vi "joystick_get_pressed.vi"(0 "JoystickDevRef 2":T2, 1 "Scaler":i8=127) -> (2 "JoystickDevRef":T2, 3 "Axes":T1, 4 "Buttons":T4, 5 "Buttons Pressed?":bool[](array[boolean]))   [LabVIEW 2013]
uses:
  <vilib>/Rock Robotics/WPI/Joystick/WPI_JoystickDevRef.ctl
  <vilib>/Rock Robotics/WPI/Joystick/WPI_JoystickDeviceEnum.ctl
  <vilib>/Rock Robotics/WPI/Joystick/WPI_JoystickButtonState.ctl
  <vilib>/Rock Robotics/WPI/Joystick/WPI_JoystickCacheOp.ctl
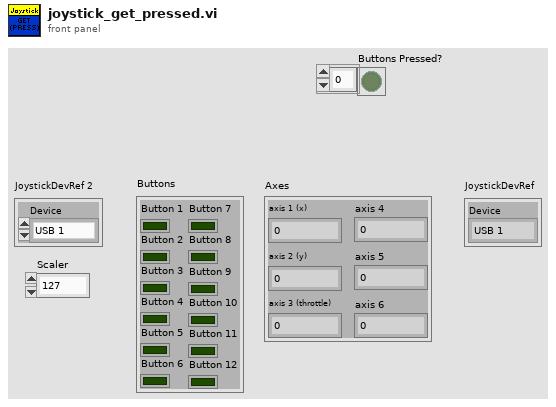
[diagram p1: front panel]
types:
  T1 = cluster{"axis 1 (x)":dbl, "axis 2 (y)":dbl, "axis 3 (throttle)":dbl, "axis 4":dbl, "axis 5":dbl, "axis 6":dbl}
  T2 = typedef "WPI_JoystickDevRef.ctl" = cluster{"Device":T3}
  T3 = typedef "WPI_JoystickDeviceEnum.ctl" = enum16{"USB 1", "USB 2", "USB 3", "USB 4", "Kinect 1", "Kinect 2"}
  T4 = typedef "WPI_JoystickButtonState.ctl" = cluster{"Button 1":bool, "Button 2":bool, "Button 3":bool, "Button 4":bool, "Button 5":bool, "Button 6":bool, "Button 7":bool, "Button 8":bool, "Button 9":bool, "Button 10":bool, "Button 11":bool, "Button 12":bool}
  T5 = cluster{"axis 1 (x)":dbl, "axis 2 (y)":dbl, "axis 3 (z)":dbl, "axis 4 (twist)":dbl, "axis 5 (throttle)":dbl, "axis 6 (num)":dbl}
  T6 = typedef "WPI_JoystickCacheOp.ctl" = enum16{"Set", "Init", "Get"}
  T7 = typedef "WPI_JoystickDeviceDataRaw.ctl" = cluster{"axis 1":i8, "axis 2":i8, "axis 3":i8, "axis 4":i8, "axis 5":i8, "axis 6":i8, "Buttons":u16}
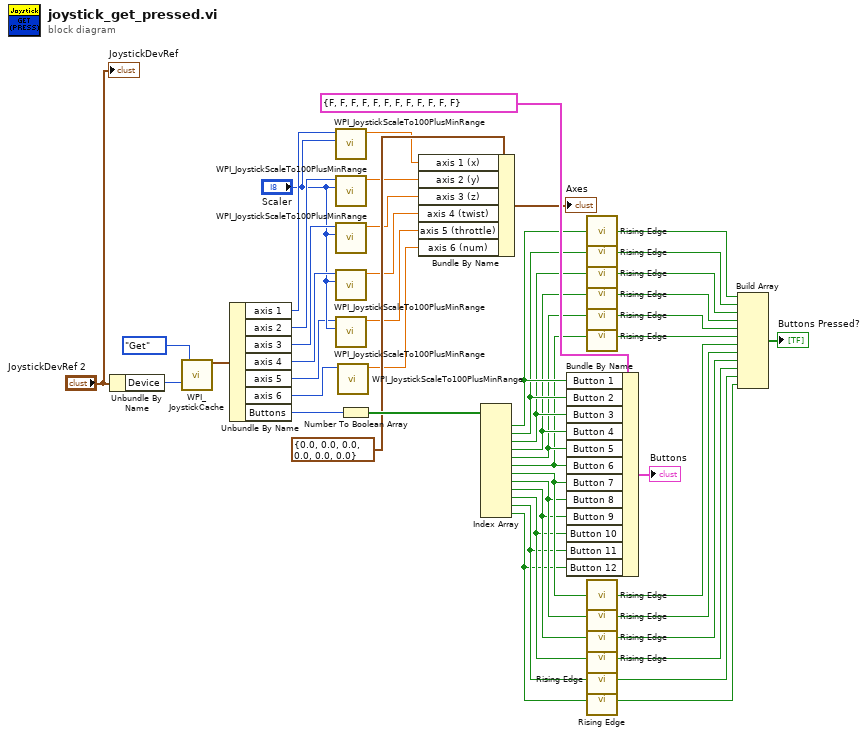
[diagram p0: block diagram]
diagram:
  n1 = Unbundle By Name("JoystickDevRef 2") -> ("Device"=w47:T3)
  n2 = call <vilib>:"WPI_JoystickCache.vi"("JoystickDevice"=w47, "JoystickCacheOp"=WPI_JoystickCacheOp."Get") -> ("JoystickOut"=w46:T7)  [unwired: 6 in, 11 out]
  n3 = Unbundle By Name(w46) -> ("axis 1"=w41:i8, "axis 2"=w40:i8, "axis 3"=w39:i8, "axis 4"=w38:i8, "axis 5"=w35:i8, "axis 6"=w36:i8, "Buttons"=w34:u16)
  n4 = call <vilib>:"WPI_JoystickScaleTo100PlusMinRange.vi"("Scaler"="Scaler", "RawValue"=w41) -> ("ScaledToPercentRange"=w31:dbl)  [unwired: 9 out]
  n5 = call <vilib>:"WPI_JoystickScaleTo100PlusMinRange.vi"("Scaler"="Scaler", "RawValue"=w40) -> ("ScaledToPercentRange"=w26:dbl)  [unwired: 9 out]
  n6 = call <vilib>:"WPI_JoystickScaleTo100PlusMinRange.vi"("Scaler"="Scaler", "RawValue"=w39) -> ("ScaledToPercentRange"=w28:dbl)  [unwired: 9 out]
  n7 = call <vilib>:"WPI_JoystickScaleTo100PlusMinRange.vi"("Scaler"="Scaler", "RawValue"=w38) -> ("ScaledToPercentRange"=w30:dbl)  [unwired: 9 out]
  n8 = call <vilib>:"WPI_JoystickScaleTo100PlusMinRange.vi"("Scaler"="Scaler", "RawValue"=w35) -> ("ScaledToPercentRange"=w27:dbl)  [unwired: 9 out]
  n9 = call <vilib>:"WPI_JoystickScaleTo100PlusMinRange.vi"("RawValue"=w36) -> ("ScaledToPercentRange"=w29:dbl)  [unwired: 10 out]
  n10 = Number To Boolean Array(number=w34) -> (Boolean array=w44:bool[])
  n11 = Bundle By Name(cluster=T5 {"axis 1 (x)"=0.0, "axis 2 (y)"=0.0, "axis 3 (z)"=0.0, "axis 4 (twist)"=0.0, "axis 5 (throttle)"=0.0, "axis 6 (num)"=0.0} ("Axes"), "axis 1 (x)"=w31, "axis 2 (y)"=w26, "axis 3 (z)"=w28, "axis 4 (twist)"=w30, "axis 5 (throttle)"=w27, "axis 6 (num)"=w29) -> (→"Axes":T5)
  n12 = Index Array(array=w44) -> (element #1=w13:bool, element #2=w12:bool, element #3=w11:bool, element #4=w10:bool, element #5=w9:bool, element #6=w8:bool, element #7=w7:bool, element #8=w6:bool, element #9=w5:bool, element #10=w4:bool, element #11=w3:bool, element #12=w2:bool)  [unwired: 12 in]
  n13 = Bundle By Name(cluster=T4 {"Button 1"=FALSE, "Button 2"=FALSE, "Button 3"=FALSE, "Button 4"=FALSE, "Button 5"=FALSE, "Button 6"=FALSE, "Button 7"=FALSE, "Button 8"=FALSE, "Button 9"=FALSE, "Button 10"=FALSE, "Button 11"=FALSE, "Button 12"=FALSE} ("Buttons"), "Button 1"=w13, "Button 2"=w12, "Button 3"=w11, "Button 4"=w10, "Button 5"=w9, "Button 6"=w8, "Button 7"=w7, "Button 8"=w6, "Button 9"=w5, "Button 10"=w4, "Button 11"=w3, "Button 12"=w2) -> (→"Buttons":T4)
  n14 = call "Rising Edge.vi"("Input"=w13) -> ("Rising Edge"=w25:bool)
  n15 = call "Rising Edge.vi"("Input"=w12) -> ("Rising Edge"=w24:bool)
  n16 = call "Rising Edge.vi"("Input"=w11) -> ("Rising Edge"=w23:bool)
  n17 = call "Rising Edge.vi"("Input"=w10) -> ("Rising Edge"=w22:bool)
  n18 = call "Rising Edge.vi"("Input"=w9) -> ("Rising Edge"=w21:bool)
  n19 = call "Rising Edge.vi"("Input"=w8) -> ("Rising Edge"=w20:bool)
  n20 = call "Rising Edge.vi"("Input"=w7) -> ("Rising Edge"=w19:bool)
  n21 = call "Rising Edge.vi"("Input"=w6) -> ("Rising Edge"=w18:bool)
  n22 = call "Rising Edge.vi"("Input"=w5) -> ("Rising Edge"=w17:bool)
  n23 = call "Rising Edge.vi"("Input"=w4) -> ("Rising Edge"=w16:bool)
  n24 = call "Rising Edge.vi"("Input"=w3) -> ("Rising Edge"=w15:bool)
  n25 = call "Rising Edge.vi"("Input"=w2) -> ("Rising Edge"=w14:bool)
  n26 = Build Array(w25, w24, w23, w22, w21, w20, w19, w18, w17, w16, w15, w14) -> (→"Buttons Pressed?":bool[])
  "JoystickDevRef" <- "JoystickDevRef 2"
